vi "FailureDescription.vi"(8 "error in (no error)":errorcluster, 10 "Actual":variant, 11 "Constraint in":refnum<class "Constraint.lvclass">) -> (0 "error out":errorcluster, 2 "Failure Description":string, 3 "Constraint out":refnum<class "Constraint.lvclass">)   [LabVIEW 2017, in "Constraint.lvlib" / "Constraint.lvclass"]
doc: "Return the second part of the scentence \"Failed asserting that ...\""
uses:
  Constraint.lvclass
  b2f06bc6-85a8-4a2f-8cfc-0c2be206f2da.vi
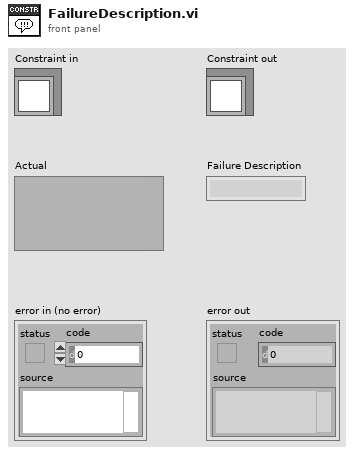
[diagram p1: front panel]
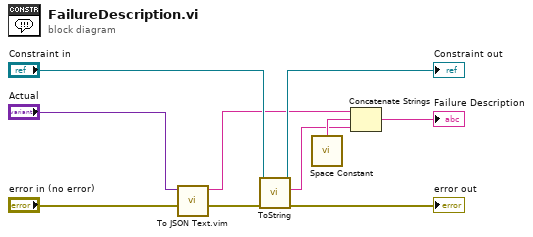
[diagram p0: block diagram]
diagram:
  n1 = call "To JSON Text.vim"("error in (no error)"="error in (no error)", "Anything"="Actual") -> ("error out"=w4:errorcluster, "<JSON>"=w2:string)  [unwired: 8 in]
  n2 = call-dynamic "ToString.vi"("error in (no error)"=w4, "Constraint in"="Constraint in") -> ("error out"=→"error out":errorcluster, "String"=w1:string, "Constraint out"=→"Constraint out":refnum<class "Constraint.lvclass">)  [unwired: 7 in]
  n3 = call <vilib>:"Space Constant.vi"() -> ("String"=w3:string)
  n4 = Concatenate Strings(w2, w3, w1) -> (→"Failure Description":string)
